vi "Dice Throws.vi"() -> (3 "Dice Out":cluster{"Dice Sum":i64, "Count":i64}[](array[cluster]))   [LabVIEW 2021]
uses:
  b5095af1-a26a-4abd-9850-73535f7e8438.vi
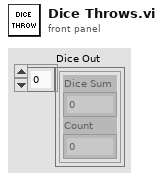
[diagram p1: front panel]
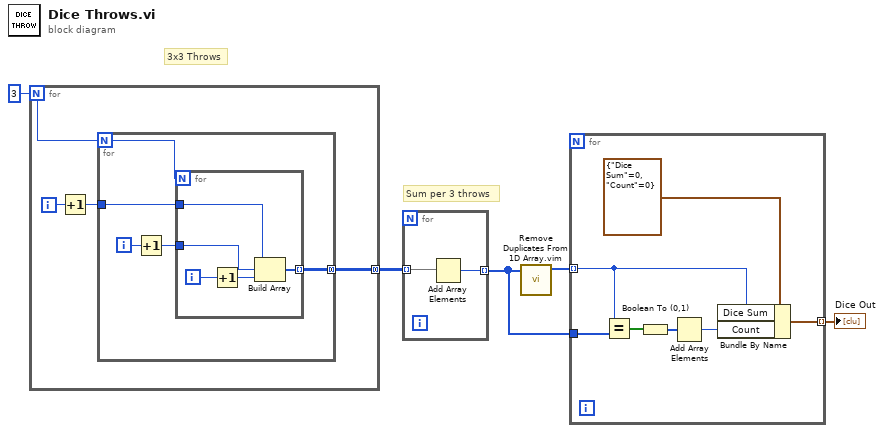
[diagram p0: block diagram]
diagram:
  # "Sum per 3 throws"
  # "3x3 Throws"
  n1 = for {
    N: 3 -> [w9]
    tunnel: [w6] -> w3 mode=concatenating
    i -> [w8]
    n2 = Increment(x=w8) -> (x+1=w7:i32)
    n3 = for {
      N: w9 -> [w14]
      tunnel: w7 -> [w13]
      tunnel: [w10] -> w6 mode=concatenating
      i -> [w12]
      n4 = Increment(x=w12) -> (x+1=w11:i32)
      n5 = for {
        N: w14 -> [_]
        tunnel: w13 -> [w18]
        tunnel: w11 -> [w17]
        tunnel: [w15] -> w10 mode=indexing
        i -> [w19]
        n6 = Increment(x=w19) -> (x+1=w16:i32)
        n7 = Build Array(w18, w17, w16) -> (w15:i32[])
      }
    }
  }
  n8 = for {
    tunnel: w3 -> [w20] mode=indexing
    tunnel: [w21] -> w2 mode=indexing
    n9 = Add Array Elements(numeric array=w20) -> (sum=w21:i32)
  }
  n10 = call "Remove Duplicates From 1D Array.vim"("array"=w2) -> ("array with duplicates removed"=w5:i32[])  [unwired: 10 in]
  n11 = for {
    tunnel: w5 -> [w23] mode=indexing
    tunnel: w2 -> [w28]
    tunnel: [w22] -> w1 mode=indexing
    n12 = Equal?(x=w23, y=w28) -> (x = y?=w27:bool[])
    n13 = Boolean To (0,1)(Boolean=w27) -> (0, 1=w26:i16[])
    n14 = Add Array Elements(numeric array=w26) -> (sum=w25:i16)
    n15 = Bundle By Name(cluster=cluster{"Dice Sum":i64, "Count":i64} {"Dice Sum"=0, "Count"=0}, "Dice Sum"=w23, "Count"=w25) -> (w22:cluster{"Dice Sum":i64, "Count":i64})
  }
  "Dice Out" <- w1
